vi "Module Pre-Loop Init.vi"(8 "error in (no error)":errorcluster, 11 "Top Level VI Ref in":refnum<vi>) -> (0 "error out":errorcluster)   [LabVIEW 2018, in "Vibration.lvlib"]
doc: "This subVI completes all initialization for communications and user events at the beginning of the top-level VI."
uses:
  Vibration.lvlib
  Private Controls/Module Data.ctl
  Private Controls/Module Action.ctl
  Private Controls/Queue Comms FGV Action.ctl
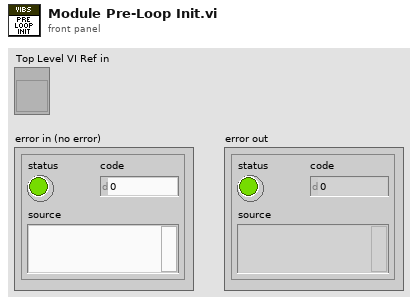
[diagram p1: front panel]
types:
  T1 = typedef "Vibration.lvlib/Queue Comms FGV Action.ctl" = enum16{"Get", "Set", "Release"}
  T2 = typedef "Vibration.lvlib/Module Data.ctl" = cluster{"Data":variant, "Action":T3}
  T3 = typedef "Vibration.lvlib/Module Action.ctl" = enum16{"Init", "Waterfall Select", "Read", "Accel Sensitivities", "Filters", "Error"}
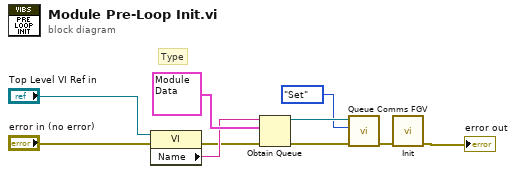
[diagram p0: block diagram]
diagram:
  # "Type"
  n1 = property class="VI"(reference="Top Level VI Ref in", error in="error in (no error)") -> (error out=w2:errorcluster, "Name"=w3:string)  [unwired: 1 out]
  n2 = Obtain Queue(name (unnamed)=w3, element data type=T2 {"Data"=variant, "Action"=enum."Init"} ("Module Data"), error in (no error)=w2) -> (queue out=w6:refnum<queue>, error out=w7:errorcluster)  [unwired: 2 in, 1 out]
  n3 = call "Queue Comms FGV.vi"("error in (no error)"=w7, "Action (Get)"=Queue_Comms_FGV_Action."Set", "Queue in"=w6) -> ("error out"=w8:errorcluster)  [unwired: 7 in, 1 out]
  n4 = call "Init.vi"("error in"=w8) -> ("error out"=→"error out":errorcluster)  [unwired: 10 in]
